vi "NIVS.Channels.Read.vi"(8 "error in (no error)":errorcluster, 11 "State Variables":T1) -> (0 "error out":errorcluster)   [LabVIEW 2015, in "Station.Execution.lvlib"]
uses:
  Station.Execution.lvlib
  Types/Main.StateVariables.ctl
  Types/Execute.UserEventRefs.ctl
  <vilib>/NI Veristand/Execution/Workspace/SystemStateRegEventRef.ctl
  <vilib>/NI Veristand/Execution/Workspace/Target State Info.ctl
  <vilib>/NI Veristand/Execution/Workspace/Target State.ctl
  <vilib>/NI Veristand/Execution/WaveformStreaming/Waveform Data Watcher Event Data (DBL).ctl
  <vilib>/NI Veristand/Execution/WaveformStreaming/WaveformStreamSpecification.ctl
  NationalInstruments.VeriStand.ClientAPI
  <vilib>/NI Veristand/Execution/Workspace/SystemStateEventRef.ctl
  <vilib>/NI Veristand/Execution/Workspace/WorkspaceAPI.ctl
  Types/UI.Object.ctl
  Types/Waveforms.Info.ctl
  <vilib>/NI Veristand/Execution/WaveformStreaming/Registered Waveform Streams Data Event Refnum (DBL).ctl
  <vilib>/NI Veristand/Execution/WaveformStreaming/WaveformDataWatcherDBL.ctl
  <vilib>/NI Veristand/Execution/WaveformStreaming/WaveformStreamingAPI.ctl
  <vilib>/Utility/miscctls.llb/LVPositionTypeDef.ctl
  <vilib>/NI Veristand/Execution/Workspace/NI VeriStand - Get Multiple Channel Values.vi
  <vilib>/NI Veristand/Execution/Workspace/NI_VS Workspace ExecutionAPI.lvlib
  <vilib>/NI Veristand/Execution/WaveformStreaming/NI_VS Waveform Streaming Interface.lvlib
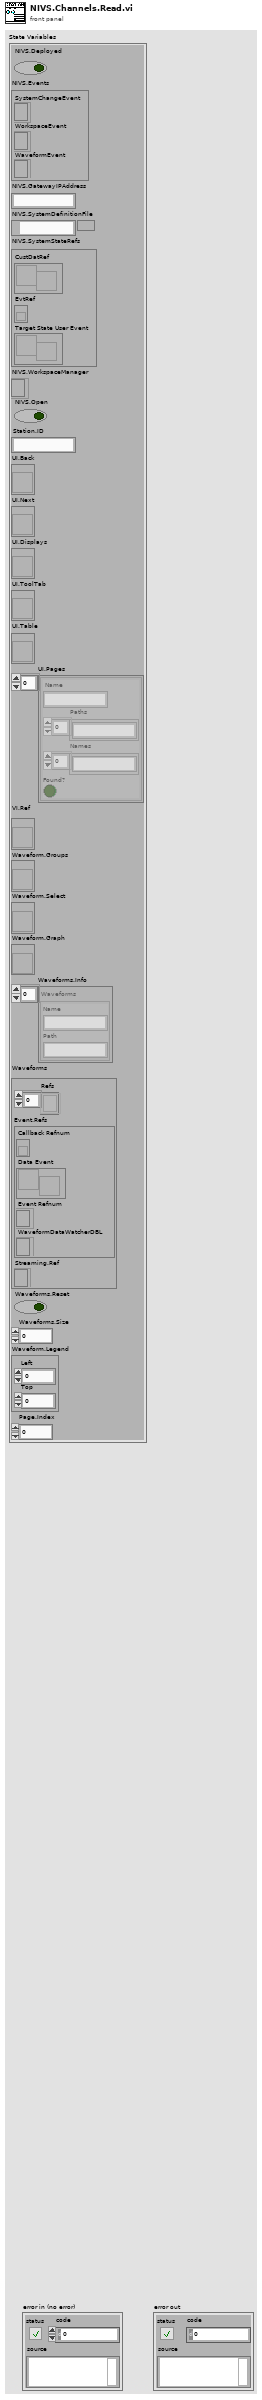
[diagram p1: front panel]
types:
  T1 = typedef "Station.Execution.lvlib/Main.StateVariables.ctl" = cluster{"NIVS.Deployed":bool, "NIVS.Events":T2, "NIVS.GatewayIPAddress":string, "NIVS.SystemDefinitionFile":path, "NIVS.SystemStateRefs":T4, "NIVS.WorkspaceManager":T5, "NIVS.Open":bool, "Station.ID":string, "UI.Back":refnum<vi>, "UI.Next":refnum<vi>, "UI.Displays":refnum<vi>, "UI.ToolTab":refnum<vi>, "UI.Table":refnum<vi>, "UI.Pages":T6[], "VI.Ref":refnum<vi>, "Waveform.Groups":refnum<vi>, "Waveform.Select":refnum<vi>, "Waveform.Graph":refnum<vi>, "Waveforms.Info":T7[], "Waveforms":cluster{"Refs":T8[], "Event.Refs":T9, "Streaming.Ref":T11}, "Waveforms.Reset":bool, "Waveforms.Size":i32, "Waveform.Legend":T12, "Page.Index":u32}
  T2 = typedef "Station.Execution.lvlib/Execute.UserEventRefs.ctl" = cluster{"SystemChangeEvent":T3, "WorkspaceEvent":refnum<event-registration>, "WaveformEvent":refnum<event-registration>}
  T3 = typedef "NI_VS Workspace ExecutionAPI.lvlib/SystemStateRegEventRef.ctl" = refnum<event-registration>
  T4 = typedef "NI_VS Workspace ExecutionAPI.lvlib/SystemStateEventRef.ctl" = cluster{"CustDatRef":refnum<user-event>, "EvtRef":refnum<k27>, "Target State User Event":refnum<user-event>}
  T5 = typedef "NI_VS Workspace ExecutionAPI.lvlib/WorkspaceAPI.ctl" = refnum<k24>
  T6 = typedef "Station.Execution.lvlib/UI.Object.ctl" = cluster{"Name":string, "Paths":string[], "Names":string[], "Found?":bool}
  T7 = typedef "Station.Execution.lvlib/Waveforms.Info.ctl" = cluster{"Name":string, "Path":string}
  T8 = typedef "NI_VS Waveform Streaming Interface.lvlib/WaveformStreamSpecification.ctl" = refnum<k24>
  T9 = typedef "NI_VS Waveform Streaming Interface.lvlib/Registered Waveform Streams Data Event Refnum (DBL).ctl" = cluster{"Callback Refnum":refnum<k27>, "Data Event":refnum<user-event>, "Event Refnum":refnum<event-registration>, "WaveformDataWatcherDBL":T10}
  T10 = typedef "NI_VS Waveform Streaming Interface.lvlib/WaveformDataWatcherDBL.ctl" = refnum<k24>
  T11 = typedef "NI_VS Waveform Streaming Interface.lvlib/WaveformStreamingAPI.ctl" = refnum<k24>
  T12 = typedef "LVPositionTypeDef.ctl" = cluster{"Left":i32, "Top":i32}
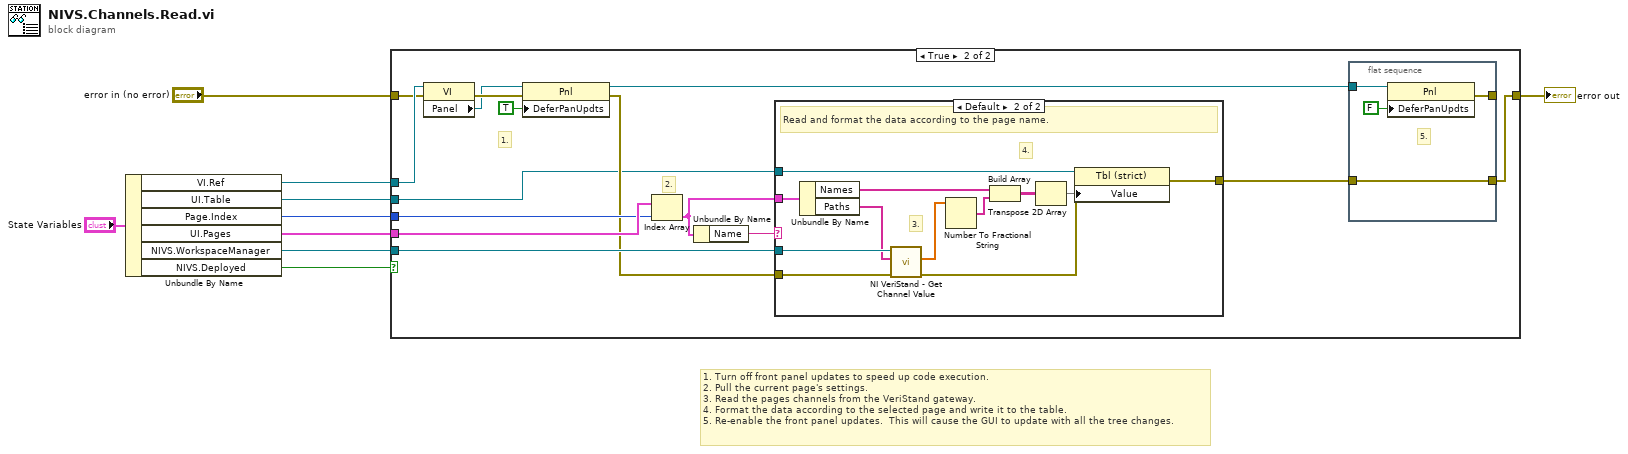
[diagram p0: block diagram]
diagram:
  # "1. Turn off front panel updates to speed up code execution.\n2. Pull the current page's settings.\n3. Read the pages channels from the VeriStand gateway.\n4. Format the data according to the selected page and write it to the table.\n5. Re-enable the front panel updates.  This will cause the GUI to update with all the tree changes."
  n1 = Unbundle By Name("State Variables") -> ("VI.Ref"=w4:refnum<vi>, "UI.Table"=w1:refnum<vi>, "Page.Index"=w3:u32, "UI.Pages"=w2:T6[], "NIVS.WorkspaceManager"=w9:T5, "NIVS.Deployed"=w8:bool)
  n2 = case shown="True" w8 {
    tunnel: "error in (no error)" -> [w10 w19]
    tunnel: w2 -> [_ w25]
    tunnel: [w10 w17] -> w7
    tunnel: w9 -> [_ w24]
    tunnel: w4 -> [_ w20]
    tunnel: w3 -> [_ w13]
    tunnel: w1 -> [_ w11]
    frame False {
    }
    frame True {
      # "2."
      # "1."
      n3 = property class="VI"(reference=w20, error in=w19) -> (error out=w22:errorcluster, "Panel"=w21:refnum<vi>)  [unwired: 1 out]
      n4 = property class="Pnl"(reference=w21, error in=w22, "DeferPanUpdts"=TRUE ("Defer Panel Updates")) -> (reference out=w16:refnum<vi>, error out=w12:errorcluster)
      n5 = Index Array(array=w25, index=w13) -> (element=w15:T6)
      n6 = Unbundle By Name(w15) -> ("Name"=w14:string)
      n7 = case shown="Default" w14 {
        tunnel: w15 -> [_ w33]
        tunnel: w12 -> [w30 w32]
        tunnel: w24 -> [_ w42]
        tunnel: [w30 w40] -> w18
        tunnel: w11 -> [_ w31]
        frame "OSCOPE" {
          # "OSCOPE page selected.  VS waveforms are handled differently.  Do nothing."
        }
        frame Default {
          # "4."
          # "3."
          # "Read and format the data according to the page name."
          n8 = Unbundle By Name(w33) -> ("Names"=w41:string[], "Paths"=w39:string[])
          n9 = call-poly <vilib>:"NI VeriStand - Get Channel Value.vi"("error in (no error)"=w32, "Channels"=w39, "WorkspaceManager in"=w42) -> ("error out"=w34:errorcluster, "Values"=w38:dbl[])  [unwired: 6 in, 1 out]
          n10 = Number To Fractional String(number=w38) -> (F-format string=w37:string[])  [unwired: 3 in]
          n11 = Build Array(w41, w37) -> (w36:string[][])
          n12 = Transpose 2D Array(2D array=w36) -> (transposed array=w35:string[][])
          n13 = property class="Tbl (strict)"(reference=w31, error in=w34, "Value"=w35) -> (error out=w40:errorcluster)  [unwired: 1 out]
        }
      }
      n14 = flat-sequence {
        tunnel: w16 -> [w29]
        tunnel: [w28] -> w17
        tunnel: w18 -> [w28]
        tunnel: [w27] -> _
        frame #0 {
          # "5."
          n15 = property class="Pnl"(reference=w29, "DeferPanUpdts"=FALSE ("Defer Panel Updates")) -> (error out=w27:errorcluster)  [unwired: 1 in, 1 out]
        }
      }
    }
  }
  "error out" <- w7
